vi "Shorting of Test Seq Program.vi"(5 "Feature List (Out)":T1(array[cluster])) -> (1 "Feature Step Enable":T1(array[cluster]), 2 "Feature Name":string[][](array[string]))   [LabVIEW 2015]
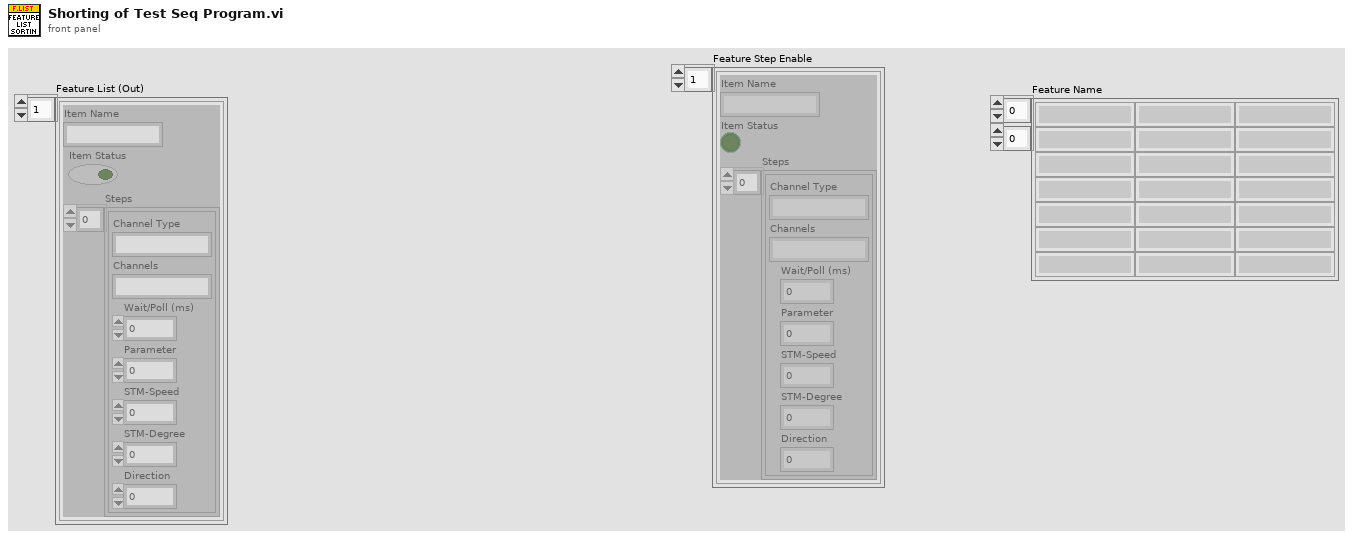
[diagram p1: front panel]
types:
  T1 = cluster{"Item Name":string, "Item Status":bool, "Steps":cluster{"Channel Type":string, "Channels":string, "Wait/Poll (ms)":u32, "Parameter":u8, "STM-Speed":i32, "STM-Degree":u32, "Direction":u8}[]}[]
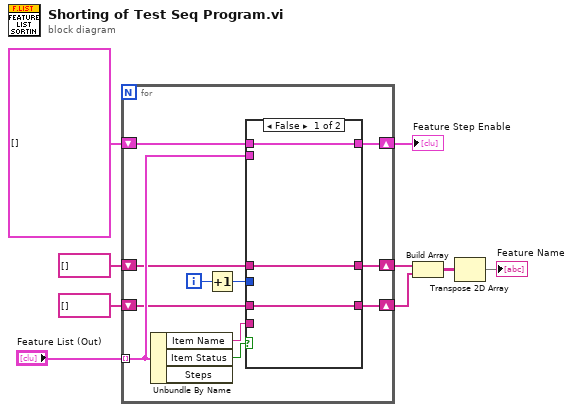
[diagram p0: block diagram]
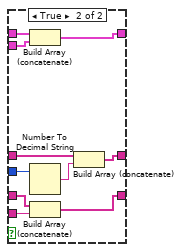
[diagram p2: hidden frame]
diagram:
  n1 = for {
    tunnel: "Feature List (Out)" -> [w18] mode=indexing
    shift-right: [w17] -> w5
    shift-left: string[] [] -> [w16]
    shift-right: [w13] -> w6
    shift-left: string[] [] -> [w12]
    shift-right: [w11] -> w4
    shift-left: T1 [] -> [w10]
    i -> [w15]
    n2 = Unbundle By Name(w18) -> ("Item Name"=w19:string, "Item Status"=w20:bool)  [unwired: 1 out]
    n3 = Increment(x=w15) -> (x+1=w14:i32)
    n4 = case shown="False" w20 {
      tunnel: w19 -> [_ w33]
      tunnel: w18 -> [_ w26]
      tunnel: [w23 w32] -> w17
      tunnel: w16 -> [w23 w31]
      tunnel: w14 -> [_ w30]
      tunnel: [w22 w28] -> w13
      tunnel: w12 -> [w22 w27]
      tunnel: [w21 w25] -> w11
      tunnel: w10 -> [w21 w24]
      frame False {
      }
      frame True {
        n5 = Build Array (concatenate)(w24, w26) -> (w25:T1)
        n6 = Number To Decimal String(number=w30) -> (decimal integer string=w29:string)  [unwired: 1 in]
        n7 = Build Array (concatenate)(w31, w33) -> (w32:string[])
        n8 = Build Array (concatenate)(w27, w29) -> (w28:string[])
      }
    }
  }
  "Feature Step Enable" <- w4
  n9 = Build Array(w6, w5) -> (w2:string[][])
  n10 = Transpose 2D Array(2D array=w2) -> (transposed array=→"Feature Name":string[][])
